vi "Add Bitfile.vi"(8 "error in (no error)":errorcluster, 10 "Engine Simulation Toolkit Bitfile":T1, 11 "EST Custom Device in":refnum<k24>) -> (0 "error out":errorcluster, 3 "EST Custom Device out":refnum<k24>)   [LabVIEW 2017, in "Engine Simulation Toolkit Scripting API.lvlib"]
uses:
  Engine Simulation Toolkit Scripting API.lvlib
  NationalInstruments.VeriStand.SystemDefinitionAPI
  Bitfile.ctl
  Shared/Properties.vi
  <vilib>/NI Veristand/Custom Device API/Set Item Property (String).vi
  Shared/Engine Simulation Toolkit Shared.lvlib
  <vilib>/NI Veristand/Custom Device API/Custom Device API.lvlib
  System Explorer/Engine Simulation Toolkit System Explorer.lvlib
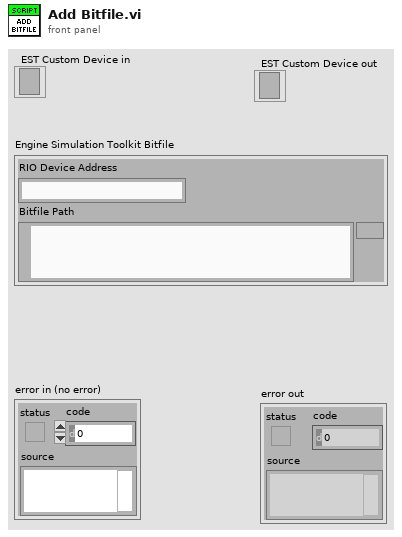
[diagram p1: front panel]
types:
  T1 = typedef "Engine Simulation Toolkit Scripting API.lvlib/Bitfile.ctl" = cluster{"RIO Device Address":string, "Bitfile Path":path}
  T2 = typedef "Custom Device API.lvlib/Custom Device Item Ref.ctl" = u64
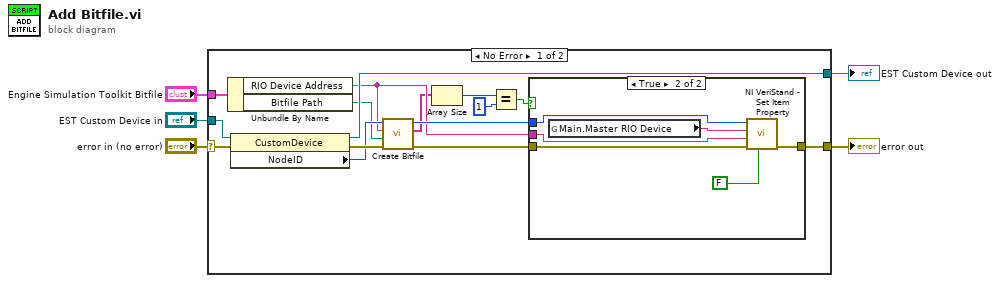
[diagram p0: block diagram]
diagram:
  n1 = case shown="No Error" "error in (no error)" {
    selector: "error in (no error)" -> [w18 w29]
    tunnel: [w14 w29] -> w5
    tunnel: "EST Custom Device in" -> [w19 w28]
    tunnel: [w13 w28] -> w2
    tunnel: "Engine Simulation Toolkit Bitfile" -> [w20 _]
    frame No Error {
      n2 = Unbundle By Name(w20) -> ("RIO Device Address"=w8:string, "Bitfile Path"=w7:path)
      n3 = property class="CustomDevice"(reference=w19, error in=w18) -> (reference out=w13:refnum<k24>, error out=w12:errorcluster, "NodeID"=w11:u64)
      n4 = call "Create Bitfile.vi"("error in (no error)"=w12, "Bitfile Path in"=w7, "RIO Device Address in"=w8, "Item Ref in"=w11) -> ("error out"=w9:errorcluster, "RIO Addresses"=w6:string[], "Item Ref out"=w10:T2)  [unwired: 5 in]
      n5 = Array Size(array=w6) -> (size(s)=w17:i32)
      n6 = Equal?(x=w17, y=1) -> (x = y?=w15:bool)
      n7 = case shown="True" w15 {
        tunnel: w9 -> [w21 w26]
        tunnel: [w21 w25] -> w14
        tunnel: w10 -> [_ w24]
        tunnel: w8 -> [_ w23]
        frame False {
        }
        frame True {
          n8 = global read "Properties.vi" "Main.Master RIO Device"() -> (w27:string)
          n9 = call-poly <vilib>:"NI VeriStand - Set Item Property.vi"("Binary String (T)"=FALSE, "error in (no error)"=w26, "Value"=w23, "Property Name"=w27, "Item Ref in"=w24) -> ("error out"=w25:errorcluster)  [unwired: 4 in, 2 out]
        }
      }
    }
    frame Error {
    }
  }
  "EST Custom Device out" <- w2
  "error out" <- w5
